vi "Get Scope Voltage Division Values.vi"(2 "error in (no error)":errorcluster) -> (0 "error out":errorcluster, 1 "Volts Per Division Values Array":dbl[](array[numeric]))   [LabVIEW 2020]
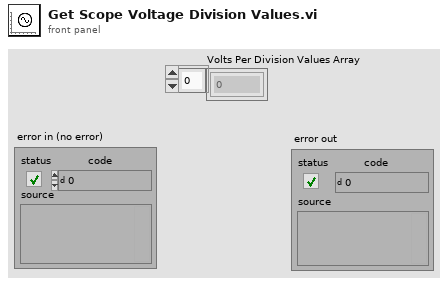
[diagram p1: front panel]
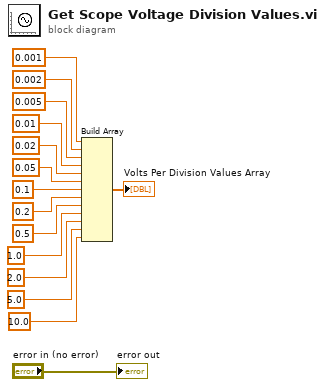
[diagram p0: block diagram]
diagram:
  n1 = Build Array(0.001, 0.002, 0.005, 0.01, 0.02, 0.05, 0.1, 0.2, 0.5, 1.0, 2.0, 5.0, 10.0) -> (→"Volts Per Division Values Array":dbl[])
  "error out" <- "error in (no error)"
